vi "Initialize Communication.vi"(0 "Session Handle in":T3, 11 "error in (no error)":errorcluster) -> (4 "Session Handle out":T3, 15 "error out":errorcluster)   [LabVIEW 2015, in "Oil.lvclass"]
uses:
  Oil.lvclass
  Typedefs/Session Handle.ctl
  <vilib>/xnet/xnet.llb/XNET Frame CAN.ctl
  <vilib>/xnet/xnet.llb/XNET Frame Type CAN.ctl
panel:
  out "Reply":T1[](array[typedef]) {"payload" format="%x"; "timestamp" format="%<%.7X\n%x>T"; "type" items=["CAN Data"=0, "CAN Remote"=1, "CAN Bus Error"=2, "J1939 Data"=192, "Delay"=224, "Log Trigger"=225, "Start Trigger"=226]; "identifier" format="%x"}
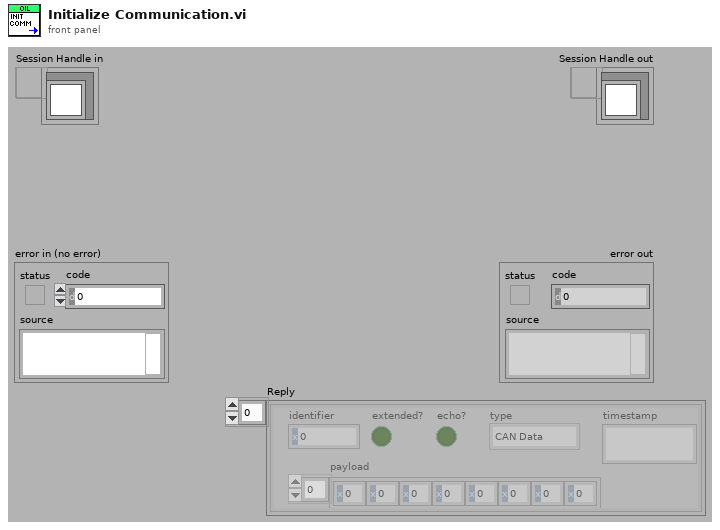
[diagram p1: front panel]
types:
  T1 = typedef "XNET Frame CAN.ctl" = cluster{"timestamp":timestamp, "payload":u8[], "identifier":u32, "type":T2, "extended?":bool, "echo?":bool}
  T2 = typedef "XNET Frame Type CAN.ctl" = u8
  T3 = typedef "Oil.lvclass/Session Handle.ctl" = refnum<data-value>
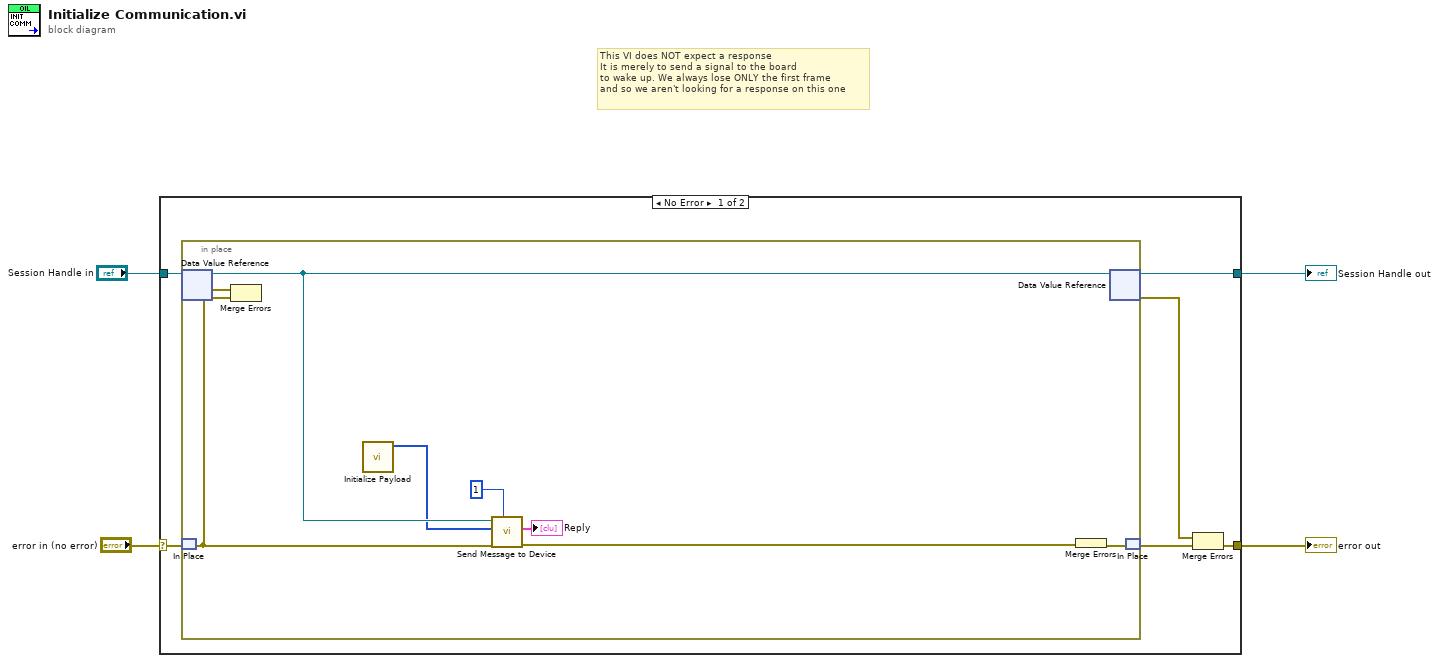
[diagram p0: block diagram]
diagram:
  # "This VI does NOT expect a response\nIt is merely to send a signal to the board\nto wake up. We always lose ONLY the first frame\nand so we aren't looking for a response on this one"
  n1 = case shown="No Error" "error in (no error)" {
    selector: "error in (no error)" -> [w5 w19]
    tunnel: "Session Handle in" -> [w10 w20]
    tunnel: [w9 w20] -> w3
    tunnel: [w6 w19] -> w2
    frame No Error {
      n2 = in-place {
        n3 = in-place-dvr #1(w10) -> (w17:refnum<class "Oil.lvclass">, w18:errorcluster)
        n4 = in-place-match #2(w5) -> (w16:errorcluster)
        n5 = Merge Errors(w16, w18) -> ()  [unwired: 1 out]
        n6 = call "Initialize Payload.vi"() -> ("Initial Payload"=w13:u8[])  [unwired: 11 in]
        n7 = call "Send Message to Device.vi"("Number of Retries"=1, "error in (no error)"=w16, "payload"=w13, "CAN Comm In"=w17) -> ("error out"=w15:errorcluster, "Reply"=→"Reply":T1[])  [unwired: 5 in, 1 out]
        n8 = Merge Errors(w15) -> (w14:errorcluster)
        n9 = in-place-dvr #1(w17) -> (w9:T3, w7:errorcluster)
        n10 = in-place-match #2(w14) -> (w8:errorcluster)
      }
      n11 = Merge Errors(w7, w8) -> (w6:errorcluster)
    }
    frame Error {
    }
  }
  "Session Handle out" <- w3
  "error out" <- w2
